vi "orc.vi"() -> ()   [LabVIEW 2009]
uses:
  <vilib>/vision/Avi1.llb/AviRefnum.ctl
  <vilib>/userDefined/High Color/IMAQdx.ctl
  <vilib>/vision/driver/NI_Vision_Acquisition_Software.lvlib
  <vilib>/vision/NI_Vision_Development_Module.lvlib
panel:
  out "Distance of Center (end)":i32
  out "Distance of Center (start)":i32
  in  "stop":bool
  in  "Camera or AVI file 2":bool
  out "IMAQ Session Out":T1 caption="Session Out"
  in  "AVI Path 2":path
  in  "Camera or AVI file":bool
  out "red orc":T2(array[cluster])
  out "red orcs":i32
  in  "Blue or Luma or Val or Inten Range 2":cluster{"Lower value":i32, "Upper value":i32}={"Lower value"=0, "Upper value"=255}
  in  "Green or Sat Range 2":cluster{"Lower value":i32, "Upper value":i32}={"Lower value"=0, "Upper value"=255}
  in  "Red or Hue Range 2":cluster{"Lower value":i32, "Upper value":i32}={"Lower value"=7, "Upper value"=14}
  in  "Select ROI":bool
  out "rectangle":i32[](array[numeric])
  in  "close":bool
  in  "Camera is blue":bool
  in  "red orc Radius":cluster{"Min Radius":sgl, "Max Radius":sgl}={"Min Radius"=8.0, "Max Radius"=50.0}
  in  "Tab Control":T3(tab)
  out "Original Image":T4(plugin-control)
  out "Orange Buoys":T4(plugin-control)
  out "Session Out":T1
  in  "Session In":T1
  in  "Avi Refnum":T5
  out "error out":errorcluster
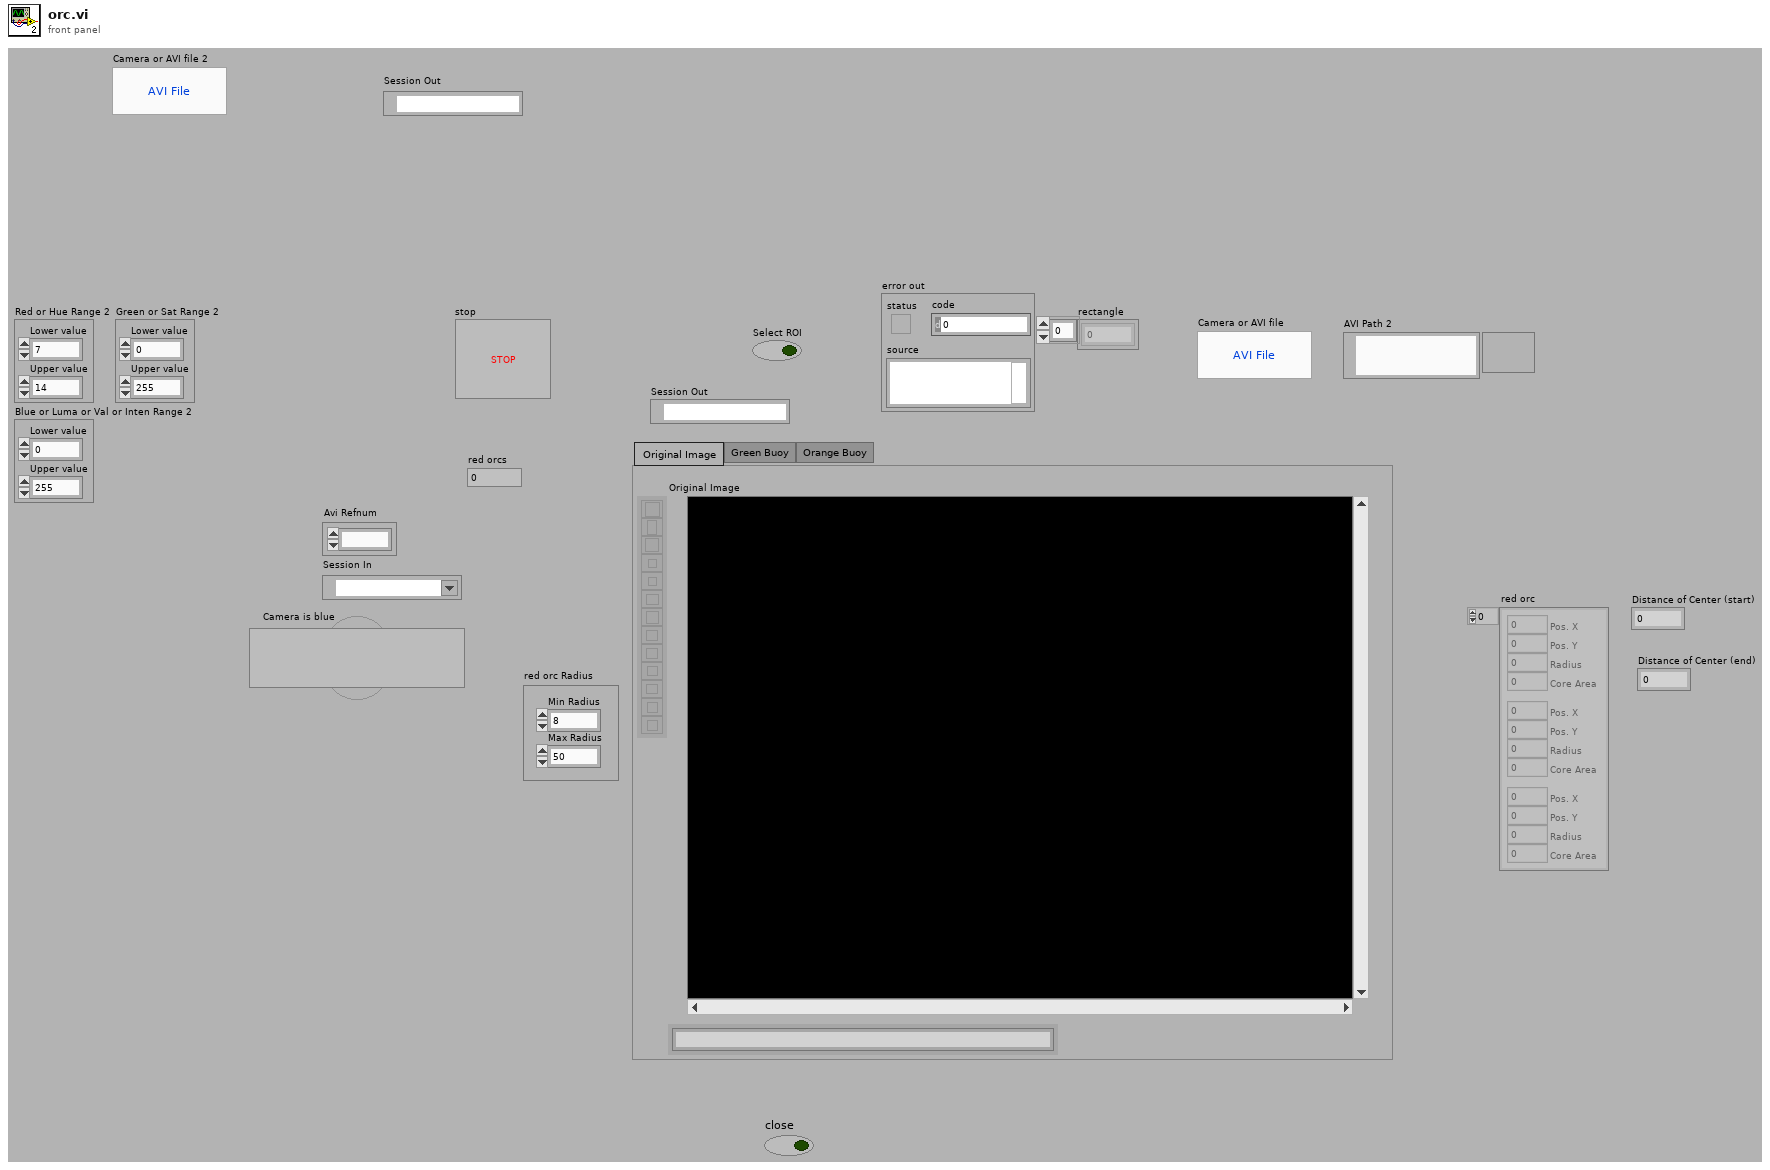
[diagram p1: front panel]
types:
  T1 = typedef "IMAQdx.ctl" = refnum<k21>
  T2 = cluster{"Pos. X":i32, "Pos. Y":i32, "Radius":i32, "Core Area":i32}[]
  T3 = enum32{"Original Image ", "Green Buoy", "Orange Buoy"}
  T4 = typedef "IMAQ Image.ctl" = refnum<image>
  T5 = typedef "AviRefnum.ctl" = refnum<k1>
  T6 = typedef "Image Type" = u32
  T7 = cluster{"Left":i32, "Top":i32, "Right":i32, "Bottom":i32}
  T8 = typedef "IMAQ Rectangle" = cluster{"Left":i32, "Top":i32, "Right":i32, "Bottom":i32, "Rotation":dbl}
  T9 = cluster{"Pos. X":i32, "Pos. Y":i32, "Radius":i32, "Core Area":i32}
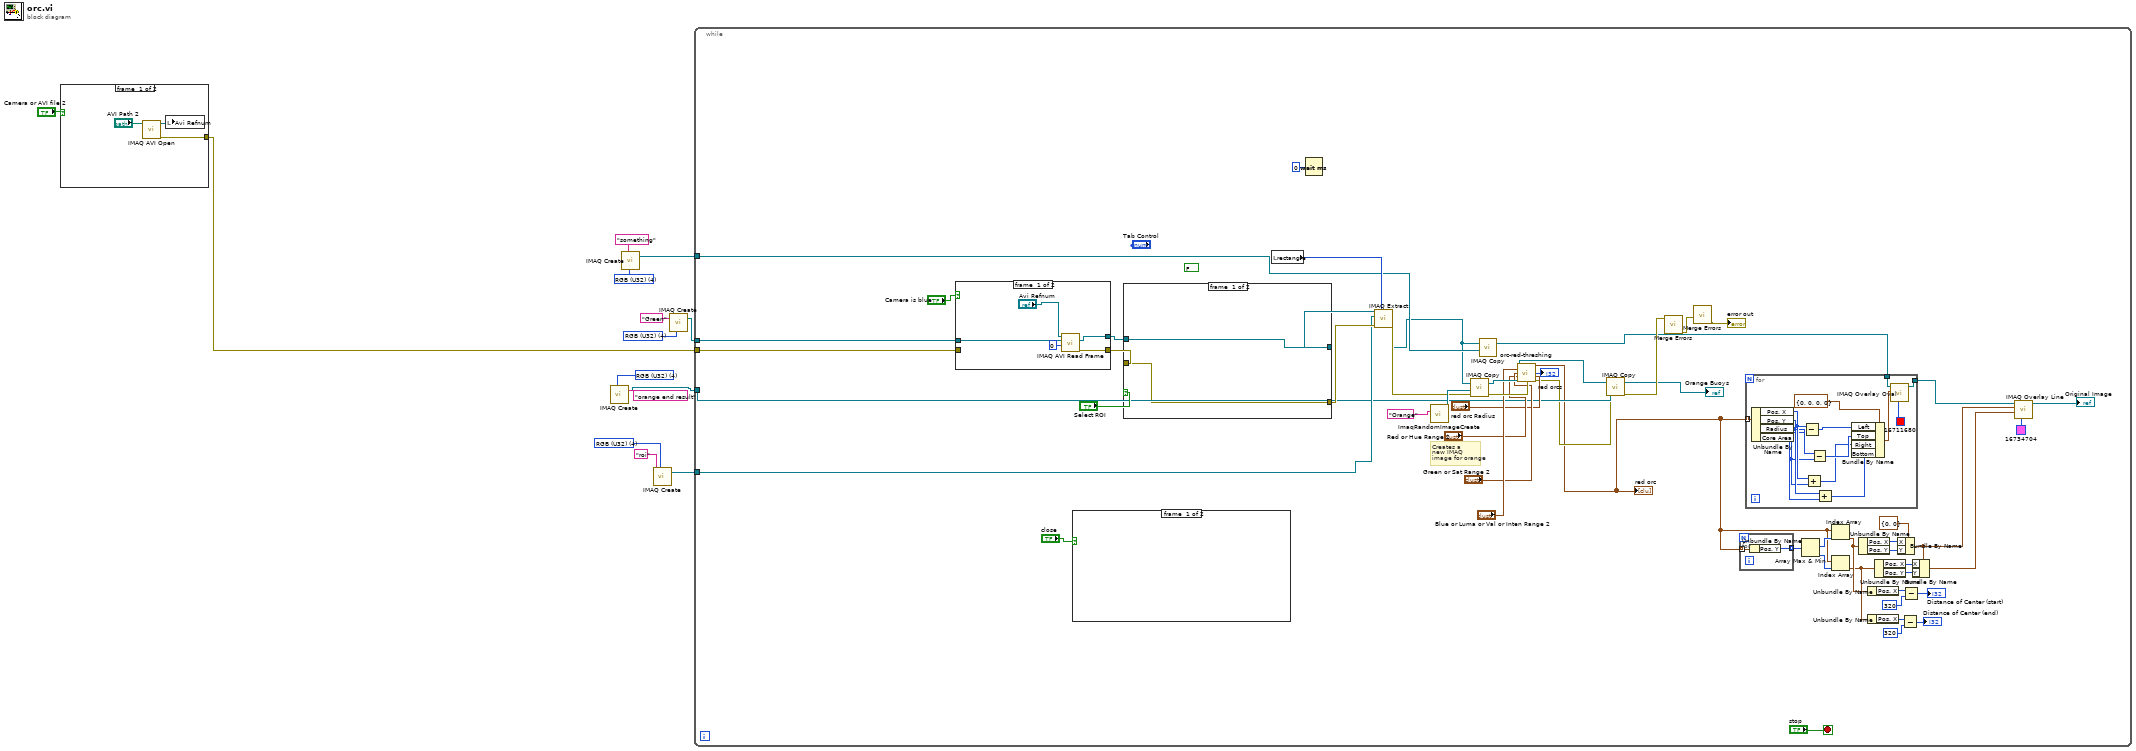
[diagram p0: block diagram]
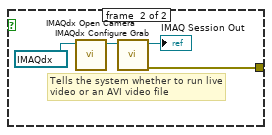
[diagram p2: hidden frame]
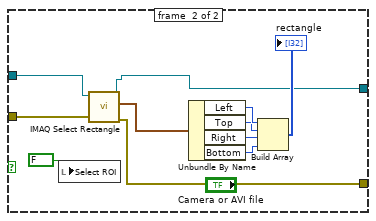
[diagram p3: hidden frame]
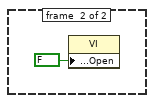
[diagram p4: hidden frame]
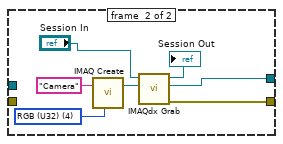
[diagram p5: hidden frame]
diagram:
  w3 = T6 4 items=["Grayscale (U8)", "Grayscale (I16)", "Grayscale (SGL)", "Complex (CSG)", "RGB (U32)", "HSL (U32)", "RGB (U64)", "Grayscale (U16)"] ("Image Type")
  w6 = T6 4 items=["Grayscale (U8)", "Grayscale (I16)", "Grayscale (SGL)", "Complex (CSG)", "RGB (U32)", "HSL (U32)", "RGB (U64)", "Grayscale (U16)"] ("Image Type")
  w9 = T6 4 items=["Grayscale (U8)", "Grayscale (I16)", "Grayscale (SGL)", "Complex (CSG)", "RGB (U32)", "HSL (U32)", "RGB (U64)"] ("Image Type")
  w12 = T6 4 items=["Grayscale (U8)", "Grayscale (I16)", "Grayscale (SGL)", "Complex (CSG)", "RGB (U32)", "HSL (U32)", "RGB (U64)", "Grayscale (U16)"] ("Image Type")
  n1 = case shown="False" "Camera or AVI file 2" {
    tunnel: [w16 w19] -> w13
    frame #0 {
      n2 = call "IMAQ AVI Open"("AVI Path"="AVI Path 2") -> ("error out"=w16:errorcluster, "Avi Refnum"=w15:T5)  [unwired: 1 in, 8 out]
      n3 = local write "Avi Refnum"(w15) -> ()
    }
    frame #1 {
      # "Tells the system whether to run live \nvideo or an AVI video file"
      n4 = call <vilib>:"IMAQdx Open Camera.vi"("Session In"=T1 "cam1") -> ("Session Out"=w21:T1)  [unwired: 2 in, 8 out]
      n5 = call <vilib>:"IMAQdx Configure Grab.vi"("Session In"=w21) -> ("error out"=w19:errorcluster, "Session Out"=→"IMAQ Session Out":T1)  [unwired: 1 in, 8 out]
    }
  }
  n6 = call "IMAQ Create"("Image Name"="orange end result", "Image Type"=w3) -> ("New Image"=w1:T4)  [unwired: 2 in, 2 out]
  n7 = call "IMAQ Create"("Image Name"="something", "Image Type"=w6) -> ("New Image"=w4:T4)  [unwired: 2 in, 2 out]
  n8 = call "IMAQ Create"("Image Name"="roi", "Image Type"=w12) -> ("New Image"=w10:T4)  [unwired: 2 in, 2 out]
  n9 = call "IMAQ Create"("Image Name"="Green", "Image Type"=w9) -> ("New Image"=w7:T4)  [unwired: 2 in, 2 out]
  n10 = while {
    tunnel: w13 -> [w53]
    tunnel: w10 -> [w50]
    tunnel: w7 -> [w49]
    tunnel: w4 -> [w48]
    tunnel: w1 -> [w46]
    stop <- "stop" stop-if-true
    (unwired) FALSE ("Maintain Size")
    # "Creates a\nnew IMAQ\nimage for orange"
    n11 = case shown="False" "Camera is blue" {
      tunnel: [w110 w114] -> w69
      tunnel: [w109 w112] -> w68
      tunnel: w53 -> [_ _]
      tunnel: w49 -> [w107 _]
      frame #0 {
        n12 = call "IMAQ AVI Read Frame"("Frame Number"=u32 0, "Image"=w107, "Avi Refnum"="Avi Refnum") -> ("error out"=w109:errorcluster, "Image Out"=w110:T4)  [unwired: 2 in, 5 out]
      }
      frame #1 {
        w116 = T6 4 items=["Grayscale (U8)", "Grayscale (I16)", "Grayscale (SGL)", "Complex (CSG)", "RGB (U32)", "HSL (U32)", "RGB (U64)"] ("Image Type")
        n13 = call "IMAQ Create"("Image Name"="Camera", "Image Type"=w116) -> ("New Image"=w115:T4)  [unwired: 2 in, 2 out]
        n14 = call <vilib>:"IMAQdx Grab.vi"("Image In"=w115, "Session In"="Session In") -> ("error out"=w112:errorcluster, "Image Out"=w114:T4, "Session Out"=→"Session Out":T1)  [unwired: 2 in, 5 out]
      }
    }
    n15 = case shown="True" "close" {
      frame #0 {
      }
      frame #1 {
        n16 = property class="VI"("Front Panel.Open"=FALSE ("Front Panel Window:Open")) -> ()  [unwired: 2 in, 2 out]
      }
    }
    n17 = case shown="True" "Select ROI" {
      tunnel: w69 -> [w93 w104]
      tunnel: w68 -> [w92 w103]
      tunnel: [w93 w94] -> w65
      tunnel: [w92 w96] -> w64
      frame #0 {
      }
      frame #1 {
        n18 = local write "Select ROI"(FALSE ("Select ROI")) -> ()
        n19 = call "IMAQ Select Rectangle"("error in (no error)"=w103, "Image In"=w104) -> ("error out"=w96:errorcluster, "Rectangle"=w102:T8, "Image Out (duplicate)"=w94:T4)  [unwired: 6 in, 1 out]
        n20 = Unbundle By Name(w102) -> ("Left"=w101:i32, "Top"=w100:i32, "Right"=w99:i32, "Bottom"=w98:i32)
        n21 = Build Array(w101, w100, w99, w98) -> (→"rectangle":i32[])
      }
    }
    n22 = local read "rectangle"() -> (w63:i32[])
    n23 = Wait (ms)(milliseconds to wait=u32 0) -> ()  [unwired: 1 out]
    n24 = call "IMAQ Extract"("Optional Rectangle"=w63, "error in (no error)"=w64, "Image Dst"=w50, "Image Src"=w65) -> ("error out"=w67:errorcluster, "Image Dst Out"=w22:T4)  [unwired: 6 in]
    n25 = call "ImaqRandomImageCreate.vi"("Image Name"="Orange") -> ("New Image"=w75:T4)  [unwired: 1 in, 9 out]
    n26 = call "IMAQ Copy"("error in (no error)"=w67, "Image Dst"=w75, "Image Src"=w22) -> ("error out"=w62:errorcluster, "Image Dst Out"=w61:T4)  [unwired: 3 out]
    n27 = call "IMAQ Copy"("Image Dst"=w48, "Image Src"=w22) -> ("Image Dst Out"=w51:T4)  [unwired: 1 in, 4 out]
    n28 = call "orc-red-threshing.vi"("Blue or Luma or Val or Inten Range"="Blue or Luma or Val or Inten Range 2", "Green or Sat Range"="Green or Sat Range 2", "Red or Hue Range"="Red or Hue Range 2", "Cluster"="red orc Radius", "Image Src"=w61, "error in (no error)"=w62) -> ("Image Out"=w60:T4, "Circles Data (calibrated)"=w33:T2, "Nb Circles"=→"red orcs":i32, "error out"=w45:errorcluster)  [unwired: 6 in]
    "red orc" <- w33
    n29 = call "IMAQ Copy"("error in (no error)"=w45, "Image Dst"=w46, "Image Src"=w60) -> ("error out"=w74:errorcluster, "Image Dst Out"=→"Orange Buoys":T4)  [unwired: 3 out]
    n30 = call <vilib>:"Merge Errors.vi"("error in 1 (no error)"=w74) -> ("error out"=w73:errorcluster)  [unwired: 3 in, 3 out]
    n31 = call <vilib>:"Merge Errors.vi"("error in 3 (no error)"=w73) -> ("error out"=→"error out":errorcluster)  [unwired: 3 in, 3 out]
    n32 = for {
      tunnel: w33 -> [w78] mode=indexing
      tunnel: [w77] -> w42 mode=indexing
      n33 = Unbundle By Name(w78) -> ("Pos. Y"=w77:i32)
    }
    n34 = for {
      tunnel: w33 -> [w91] mode=indexing
      tunnel: w51 -> [w80]
      tunnel: [w79] -> w44
      n35 = Unbundle By Name(w91) -> ("Pos. X"=w86:i32, "Pos. Y"=w85:i32, "Radius"=w83:i32)  [unwired: 1 out]
      n36 = Subtract(x=w86, y=w83) -> (x-y=w88:i32)
      n37 = Add(x=w86, y=w83) -> (x+y=w84:i32)
      n38 = Subtract(x=w85, y=w83) -> (x-y=w87:i32)
      n39 = Add(x=w85, y=w83) -> (x+y=w82:i32)
      n40 = Bundle By Name(cluster=T7 {"Left"=0, "Top"=0, "Right"=0, "Bottom"=0} ("Bounding Rectangle"), "Left"=w88, "Top"=w87, "Right"=w84, "Bottom"=w82) -> (w89:T7)
      n41 = call "IMAQ Overlay Oval"("Color"=u32 16711680, "Bounding Rectangle"=w89, "Image"=w80) -> ("Image Out"=w79:T4)  [unwired: 7 in, 1 out]
    }
    n42 = Array Max & Min(array=w42) -> (max index (indices)=w38:i32, min index (indices)=w34:i32)  [unwired: 2 out]
    n43 = Index Array(array=w33, index=w38) -> (element=w30:T9)
    n44 = Index Array(array=w33, index=w34) -> (element=w27:T9)
    n45 = Unbundle By Name(w30) -> ("Pos. X"=w36:i32, "Pos. Y"=w35:i32)
    n46 = Unbundle By Name(w30) -> ("Pos. X"=w26:i32)
    n47 = Unbundle By Name(w27) -> ("Pos. X"=w25:i32)
    n48 = Unbundle By Name(w27) -> ("Pos. X"=w32:i32, "Pos. Y"=w31:i32)
    n49 = Bundle By Name(cluster=cluster{"X":i32, "Y":i32} {"X"=0, "Y"=0} ("Start Point"), "X"=w36, "Y"=w35) -> (w37:cluster{"X":i32, "Y":i32})
    n50 = Subtract(x=w25, y=320 ("x")) -> (x-y=→"Distance of Center (end)":i32)
    n51 = Subtract(x=w26, y=320 ("x")) -> (x-y=→"Distance of Center (start)":i32)
    n52 = Bundle By Name(cluster=w37, "X"=w32, "Y"=w31) -> (w40:cluster{"X":i32, "Y":i32})
    n53 = call "IMAQ Overlay Line"("Color"=u32 16734704, "End Point"=w40, "Start Point"=w37, "Image"=w44) -> ("Image Out"=→"Original Image":T4)  [unwired: 6 in, 1 out]
  }
